vi "Finding Device in System LV2012 NIVerified.vi"() -> ()   [LabVIEW 2012]
uses:
  <resource>/objmgr/daqmx.rc
panel:
  out "Array":string[](array[string])
  out "concatenated string":string
  # "Overview\n This VI demonstrates how to use property nodes to poll your system for a particular device, so that you can programmatically choose the Physical Channel input for DAQmx Create Channel.vi.\n Requirements\n   Software\n   LabVIEW 2012 or compatible\n   NI-DAQmx 9.5.5 or compatible\n   Hardware\n   NI Multifunction DAQ Device.\n Instructions\n  1.Build up DAQ device.\n  2.Downlad and run the VI."
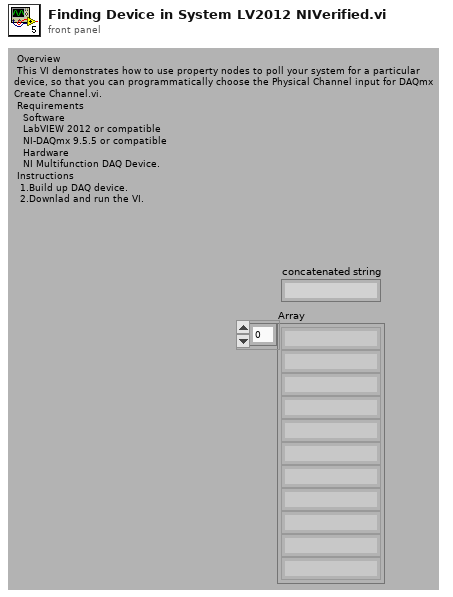
[diagram p1: front panel]
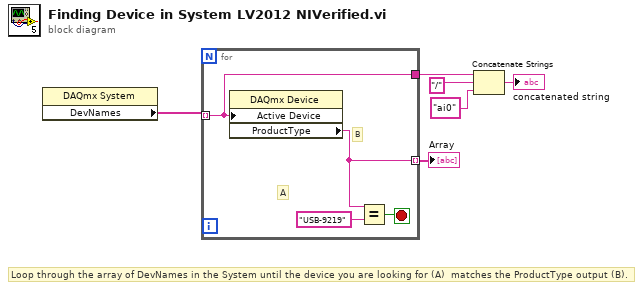
[diagram p0: block diagram]
diagram:
  # "Loop through the array of DevNames in the System until the device you are looking for (A)  matches the ProductType output (B)."
  n1 = property class="DAQmx System"() -> ("DevNames"=w6:tag[])  [unwired: 2 in, 2 out]
  n2 = for {
    tunnel: w6 -> [w10] mode=indexing
    tunnel: [w8] -> w1 mode=indexing
    tunnel: [w10] -> w5
    stop <- w9 stop-if-true
    # "B"
    # "A"
    n3 = property class="DAQmx Device"("Active Device"=w10) -> ("ProductType"=w8:string)  [unwired: 2 in, 2 out]
    n4 = Equal?(x=w8, y="USB-9219") -> (x = y?=w9:bool)
  }
  "Array" <- w1
  n5 = Concatenate Strings(w5, "/" ("string"), "ai0" ("string")) -> (→"concatenated string":string)
